vi "increment error.vi"(8 "error in (no error)":errorcluster, 11 "MB_TCP in":refnum<class "MB_TCP.lvclass">) -> (0 "error out":errorcluster, 2 "N errors":i32, 3 "MB_TCP out":refnum<class "MB_TCP.lvclass">)   [LabVIEW 2021, in "MB_TCP.lvclass"]
uses:
  MB_TCP.lvclass
  MB_TCP.lvclass/MB_TCP.ctl
  Eth Status/Eth Status.lvlib
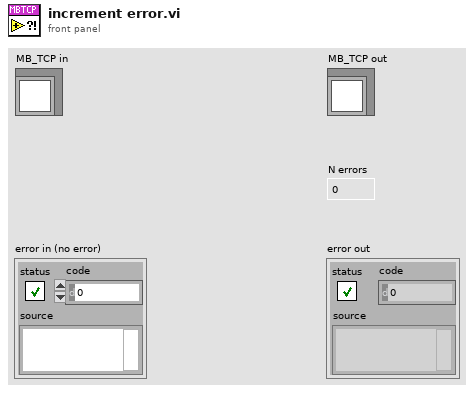
[diagram p1: front panel]
types:
  T1 = typedef "Eth Status.lvlib/Status.ctl" = cluster{"Set_states":refnum<queue>[], "WrEn":refnum<data-value>, "errors":refnum<data-value>, "connect":refnum<data-value>, "state":refnum<data-value>}
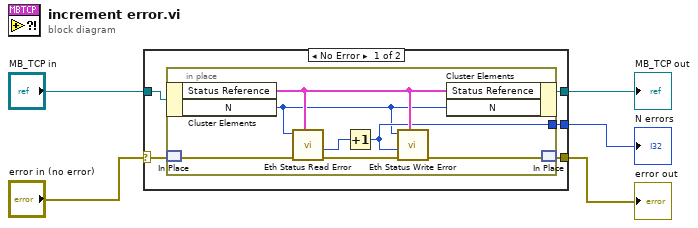
[diagram p0: block diagram]
diagram:
  n1 = case shown="No Error" "error in (no error)" {
    selector: "error in (no error)" -> [w9 w18]
    tunnel: [w8 w18] -> w1
    tunnel: [w6 w19] -> w4
    tunnel: "MB_TCP in" -> [w10 w19]
    tunnel: [w7 _] -> w2
    frame No Error {
      n2 = in-place {
        in-place-border: [w13] -> w7
        n3 = in-place-cluster #1(w10) -> ("Status Reference"=w16:T1, "N"=w11:i32)
        n4 = in-place-match #2(w9) -> (w17:errorcluster)
        n5 = call "Eth Status Read Error.vi"("Status Reference"=w16, "error in (no error)"=w17, "N"=w11) -> ("error out"=w15:errorcluster, "Error"=w14:i32)  [unwired: 7 in]
        n6 = Increment(x=w14) -> (x+1=w13:i32)
        n7 = call "Eth Status Write Error.vi"("Status Reference"=w16, "error in (no error)"=w15, "Errors"=w13, "N"=w11) -> ("error out"=w12:errorcluster)  [unwired: 7 in]
        n8 = in-place-cluster #1("Status Reference"=w16, "N"=w11) -> (w6:refnum<class "MB_TCP.lvclass">)
        n9 = in-place-match #2(w12) -> (w8:errorcluster)
      }
    }
    frame Error {
    }
  }
  "error out" <- w1
  "MB_TCP out" <- w4
  "N errors" <- w2
